vi "subVI DCR3 Lamp ShutterOnOff.vi"(1 "Lamp":bool, 2 "VISA resource name":refnum<visa-resource-name>="COM7") -> (0 "dup VISA resource name":refnum<visa-resource-name>="COM7")   [LabVIEW 2012]
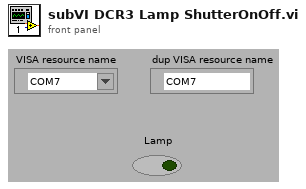
[diagram p1: front panel]
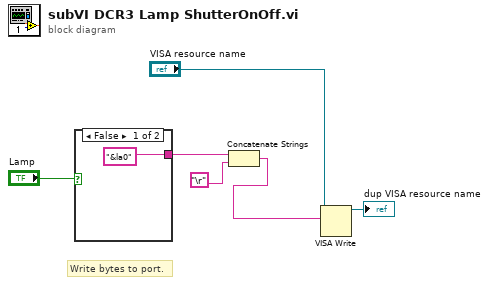
[diagram p0: block diagram]
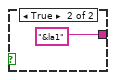
[diagram p2: hidden frame]
diagram:
  # "Write bytes to port."
  n1 = case shown="False" "Lamp" {
    tunnel: ["&la0" ("write buffer") "&la1" ("write buffer")] -> w6
    frame False {
    }
    frame True {
    }
  }
  n2 = Concatenate Strings(w6, "\r") -> (w4:string)
  n3 = VISA Write(VISA resource name="VISA resource name", write buffer=w4) -> (VISA resource name out=→"dup VISA resource name":refnum<visa-resource-name>)  [unwired: 1 in, 2 out]
